vi "Disconnect Channels (Single).vi"(8 "error in (no error)":errorcluster, 9 "channel 2":string, 10 "channel 1":string, 11 "session in":T1) -> (0 "error out":errorcluster, 3 "session out":T1)   [LabVIEW 2020, in "SLSC Switch.lvlib"]
doc: "Breaks the path between two channels created with the SLSC Switch.lvlib:Connect Channels or the SLSC Switch.lvlib:Set Path. If no connection exists between the channels, NI-SLSC Switch returns an error."
uses:
  <vilib>/SLSC_Switch/SLSC Switch.lvlib
  nislscsl.dll
  <vilib>/userdefined/High Color/SLSC_Switch/nislscslSession.ctl
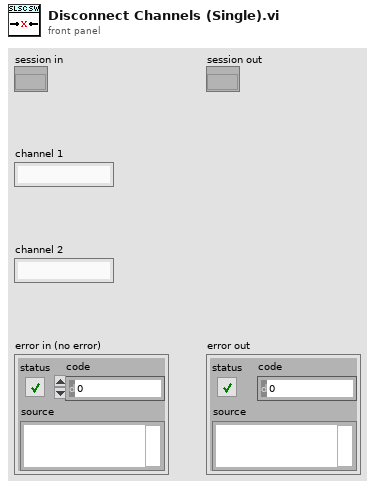
[diagram p1: front panel]
types:
  T1 = typedef "nislscslSession.ctl" = refnum<k20>
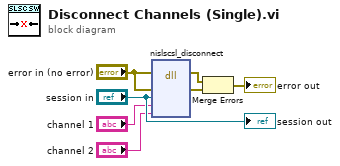
[diagram p0: block diagram]
diagram:
  n1 = dll-call lib="nislscsl.*" fn="nislscsl_disconnect"(error in="error in (no error)", "errorCluster"="error in (no error)", "sessionHandle"="session in", "channel1"="channel 1", "channel2"="channel 2") -> (error out=w7:errorcluster, "errorCluster"=w6:errorcluster)  [unwired: 6 in, 1 out]
  n2 = Merge Errors(w7, w6) -> (→"error out":errorcluster)
  "session out" <- "session in"
